vi "Cluster_Analysis.vi"(8 "Shift In":T7[](array[typedef]), 10 "Time Trace in":T6[](array[typedef]), 11 "Analysis Info cluster":T2[](array[typedef]) {"Kurt_u" format="%_3g"; "u^4" format="%_3g"; "u^3" format="%_3g"; "Sd Error in Variance" format="%_3g"; "u^2" format="%_3g"; "Sd Error in Mean" format="%_3g"; "U" format="%_3g"; "Sync Delay Time (s)" format="%.4f"; "Total Meas Time (s)" format="%_5g"; "Skew_u" format="%_3g"; "% u'/U" format="%_3g"}) -> (0 "Shift Out":T7[](array[typedef]), 1 "Autocorrelation":T1[](array[typedef]) {"X array" format="%^_5g"; "Y array" format="%^_5g"}, 2 "Histogram":T1[](array[typedef]) {"X array" format="%^_5g"; "Y array" format="%^_5g"}, 3 "Analysis Info Cluster Out":T2[](array[typedef]) {"Kurt_u" format="%_3g"; "u^4" format="%_3g"; "u^3" format="%_3g"; "Sd Error in Variance" format="%_3g"; "u^2" format="%_3g"; "Sd Error in Mean" format="%_3g"; "U" format="%_3g"; "Sync Delay Time (s)" format="%.4f"; "Total Meas Time (s)" format="%_5g"; "Skew_u" format="%_3g"; "% u'/U" format="%_3g"}, 4 "Spectra":T1[](array[typedef]) {"X array" format="%^_5g"; "Y array" format="%^_5g"}, 5 "Error String":string)   [LabVIEW 2022 SP3]
uses:
  Controls/Shift_Cluster.ctl
  Controls/Time_Trace_Cluster.ctl
  Controls/Analysis_info_cluster.ctl
  Controls/Inst_type.ctl
  Controls/Instrument_Array.ctl
  Controls/channelState.ctl
  Controls/XY_Plot_Cluster.ctl
  FFID/FFID Calib Constants index.ctl
  Globals/Meas_global.vi
  Globals/LDA_global.vi
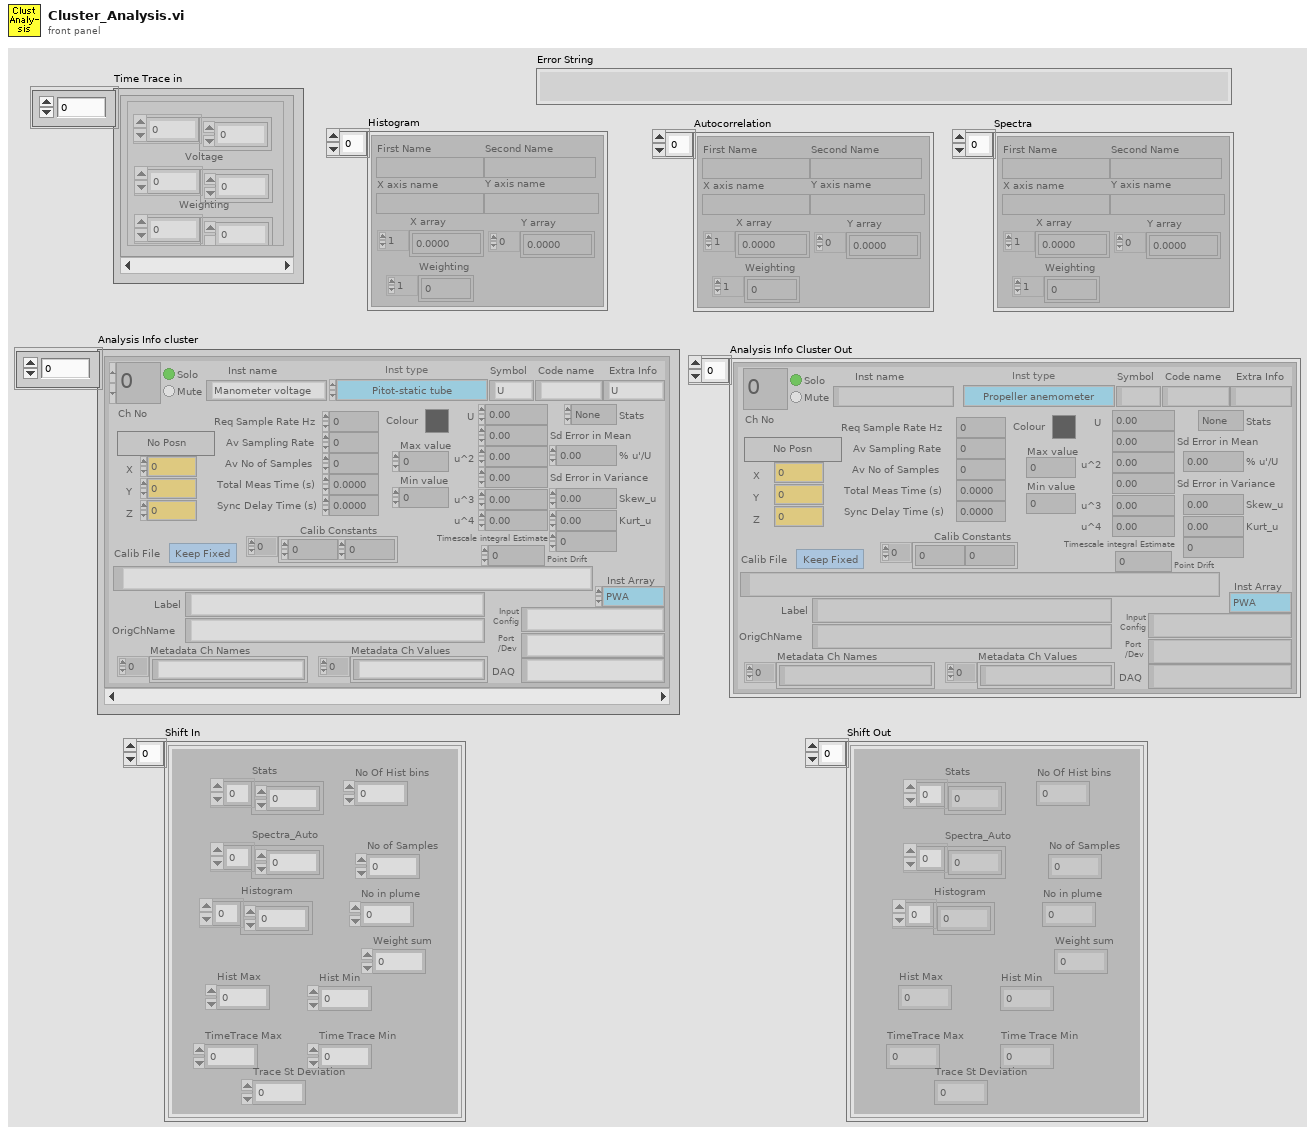
[diagram p1: front panel]
types:
  T1 = typedef "XY_Plot_Cluster.ctl" = cluster{"First Name":string, "Second Name":string, "X axis name":string, "Y axis name":string, "X array":dbl[], "Y array":dbl[], "Weighting":dbl[]}
  T2 = typedef "Analysis_info_cluster.ctl" = cluster{"Colour":u32, "Inst type":T3, "Inst name":string, "Symbol":string, "Code name":string, "Extra Info":string, "Inst Array":T4, "U":dbl, "u^2":dbl, "u^3":dbl, "u^4":dbl, "Skew_u":dbl, "Kurt_u":dbl, "Sd Error in Mean":dbl, "% u'/U":dbl, "X":dbl, "Y":dbl, "Z":dbl, "Timescale integral Estimate":dbl, "Sd Error in Variance":dbl, "Calib File":path, "Calib Constants":dbl[], "Output Position":bool, "Stats":enum16{"None", "Basic", "Full"}, "Av Sampling Rate":dbl, "Av No of Samples":dbl, "Total Meas Time (s)":dbl, "OrigChName":string, "Max value":dbl, "Min value":dbl, "Req Sample Rate Hz":dbl, "Sync Delay Time (s)":dbl, "Ch No":i16, "Device":string, "Use Latest Calib":bool, "Port":string, "Metadata Ch Names":string[], "Metadata Ch Values":string[], "Label":string, "chState":T5, "Point Drift":dbl, "inputConfig":string}
  T3 = typedef "Inst_type.ctl" = enum16{"Raw voltage", "Raw with zero offsetting", "Propeller anemometer", "Pressure Transducer", "Pitot-static tube", "Hot wire", "Cross wire 1", "Cross wire 2", "Generic Linear", "Generic Polynomial", "Generic BackPoly", "Fast FID", "Thermocouple", "Cold wire", "Pulsed Wire", "LDA Vel", "LDA Tran time", "LDA Arr time", "Microphone"}
  T4 = typedef "Instrument_Array.ctl" = enum16{"PWA", "LDA", "Analogue"}
  T5 = typedef "channelState.ctl" = enum32{"No Selection", "Solo", "Mute"}
  T6 = typedef "Time_Trace_Cluster.ctl" = cluster{"Weighting":dbl[], "Voltage":dbl[], "Eng Values":dbl[]}
  T7 = typedef "Shift_Cluster.ctl" = cluster{"Stats":dbl[], "Spectra_Auto":dbl[], "Histogram":dbl[], "Hist Max":dbl, "Hist Min":dbl, "No of Samples":i32, "No in plume":i32, "Weight sum":dbl, "No Of Hist bins":i32, "TimeTrace Max":dbl, "Time Trace Min":dbl, "Trace St Deviation":dbl}
  T8 = typedef "FFID Calib Constants index.ctl" = u16
  T9 = typedef "LDA_Channel.ctl" = cluster{"Wavelength (nm)":dbl, "Vel Comp":string, "Max Velocity":dbl, "Min Velocity":dbl, "Max Record length":u16, "Signal gain (dB)":i16, "High voltage":i16, "Optics Conversion Factor":dbl, "Min Record length":u16, "Multiply Velocity by -1":bool, "Signal to Noise Ratio":string, "Validation Ratio":string, "Probe":string, "Laser":string, "BSA":string, "Lense":string, "Beam Separation (mm)":dbl, "Focal Length (mm)":dbl, "COLOUR":u32, "BSA IP":string, "Velocity Range (m/s)":dbl, "Centre Velocity (m/s)":dbl, "Unshifted mW":dbl, "Shifted mW":dbl, "Bandwidth Hz":dbl, "Req Sampling Rate Hz":dbl, "Ch":i32, "CenterFreq Hz":dbl, "Laser IP":string, "Sync Delay (s)":dbl}
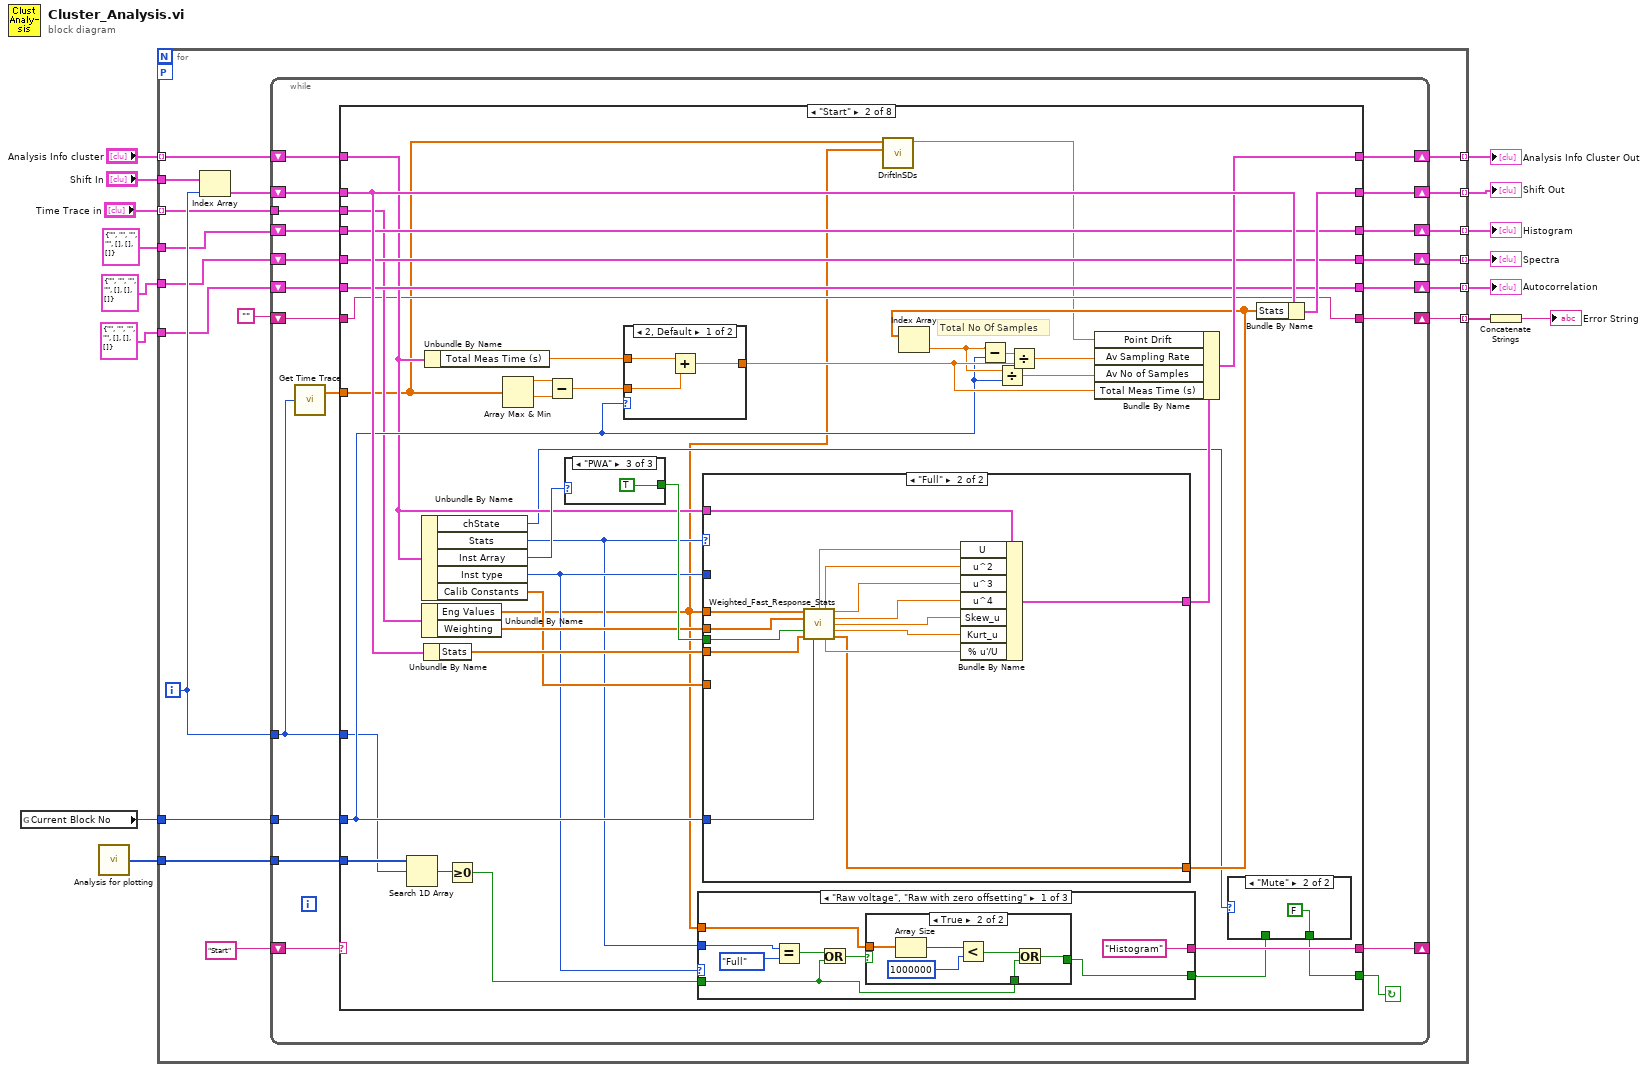
[diagram p0: block diagram]
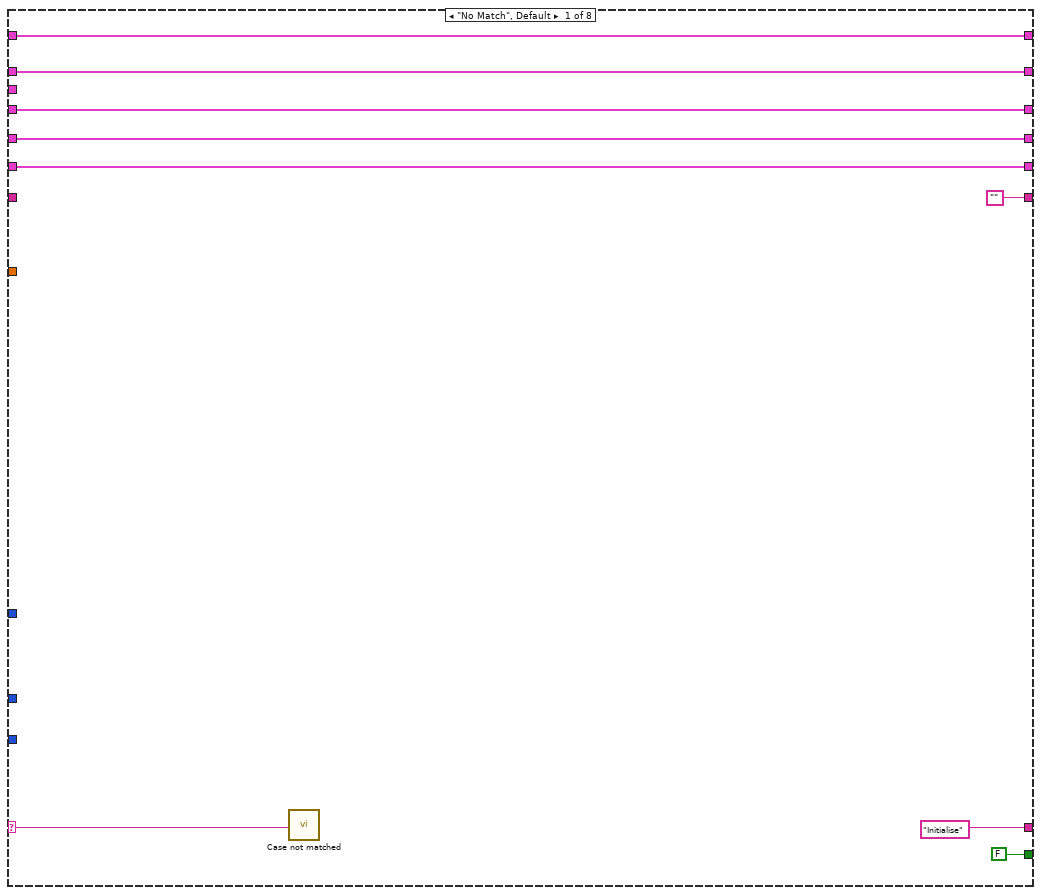
[diagram p2: hidden frame]
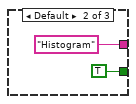
[diagram p5: hidden frame]
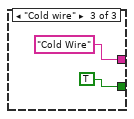
[diagram p6: hidden frame]
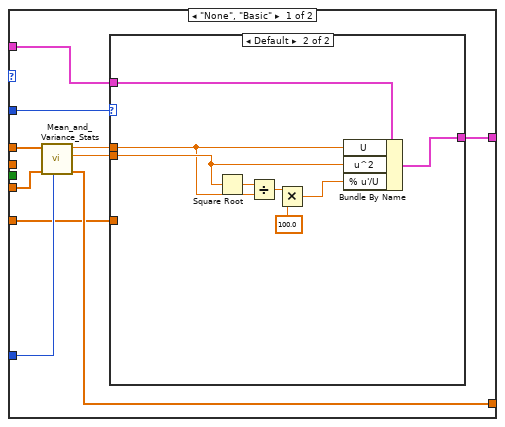
[diagram p8: hidden frame]
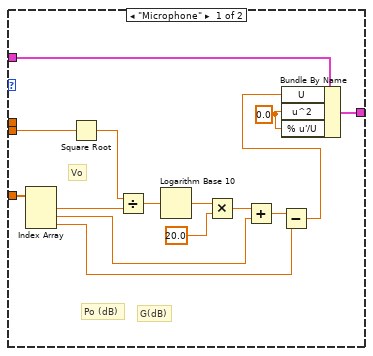
[diagram p9: hidden frame]
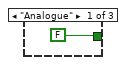
[diagram p10: hidden frame]
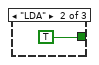
[diagram p11: hidden frame]
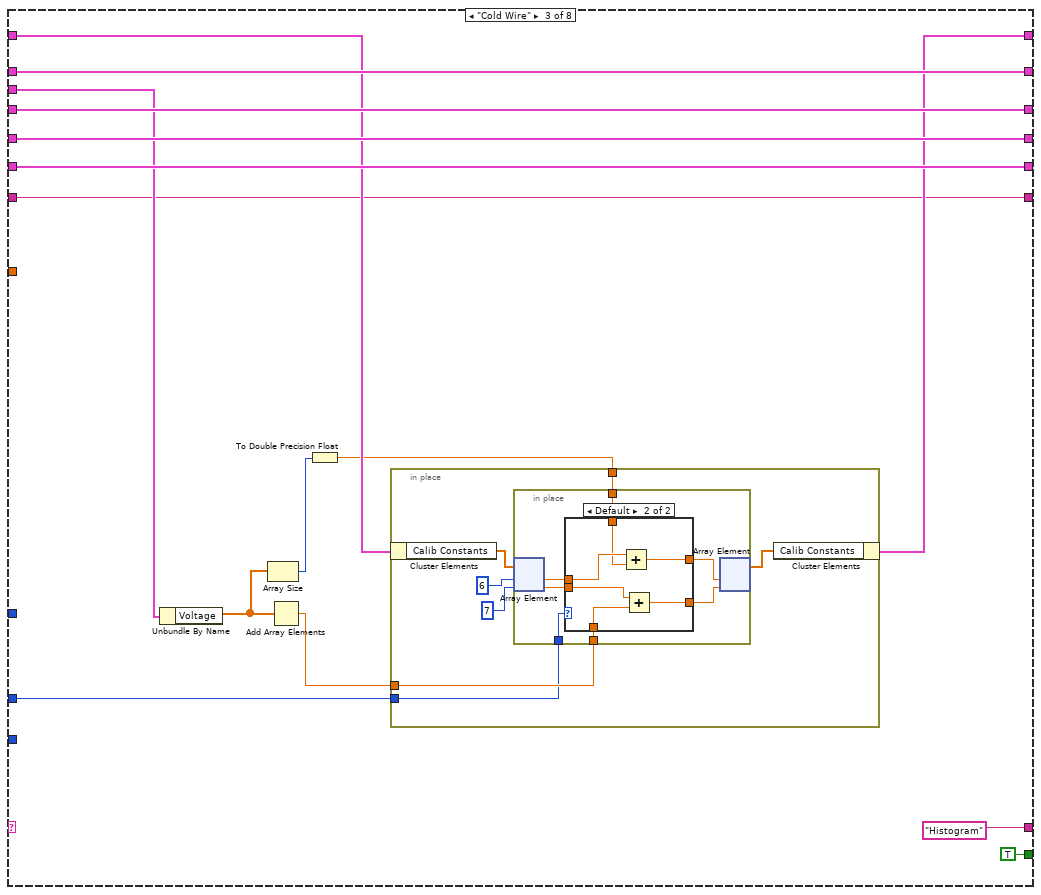
[diagram p12: hidden frame]
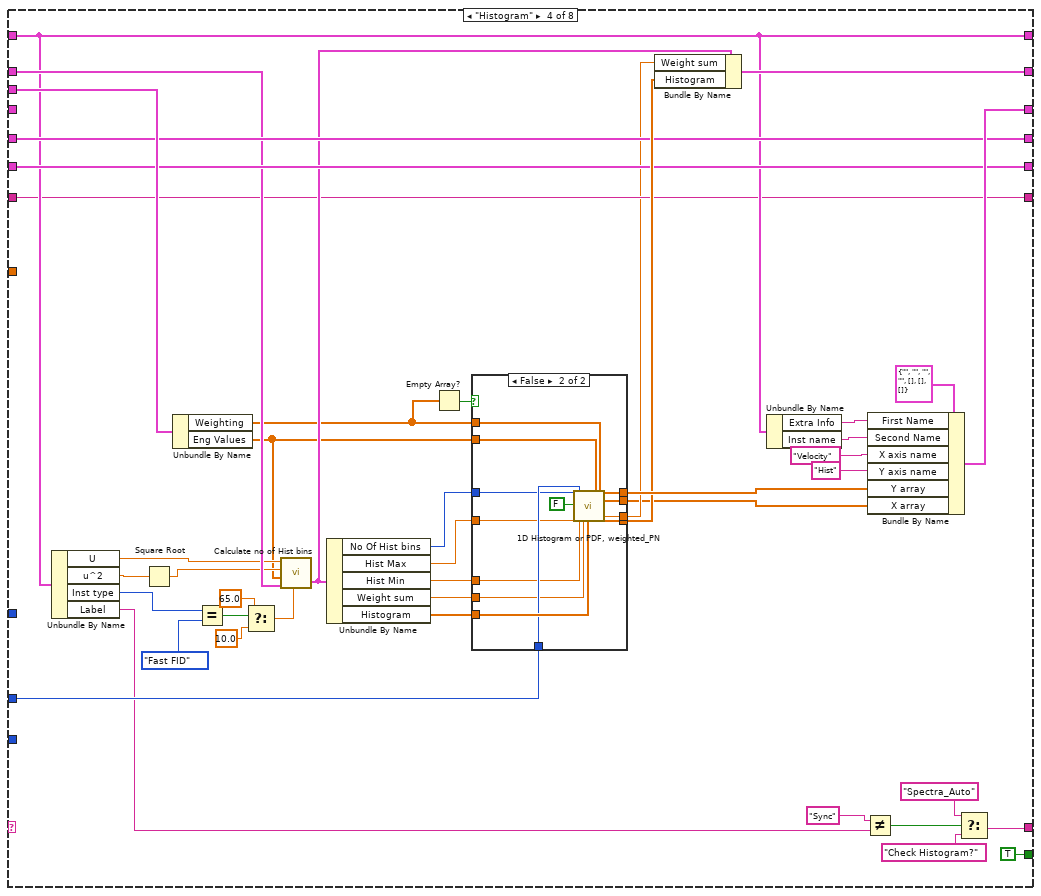
[diagram p14: hidden frame]
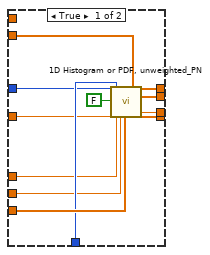
[diagram p15: hidden frame]
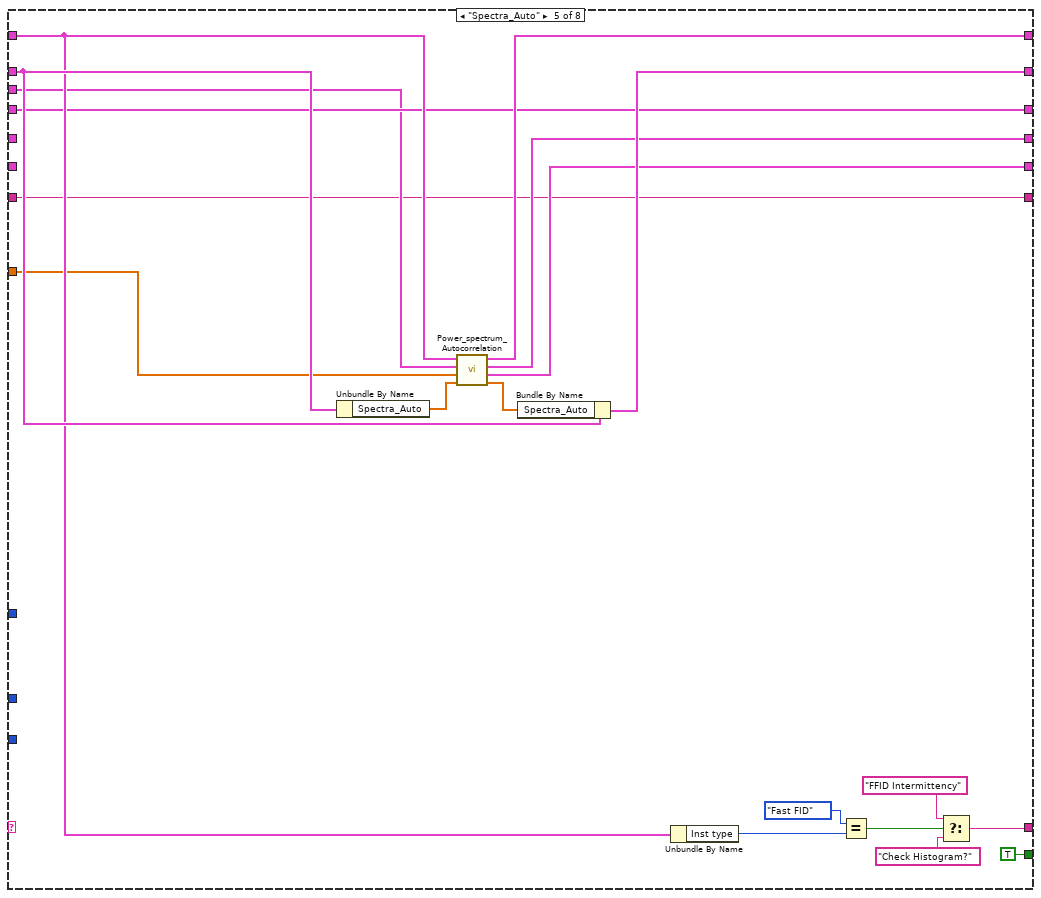
[diagram p16: hidden frame]
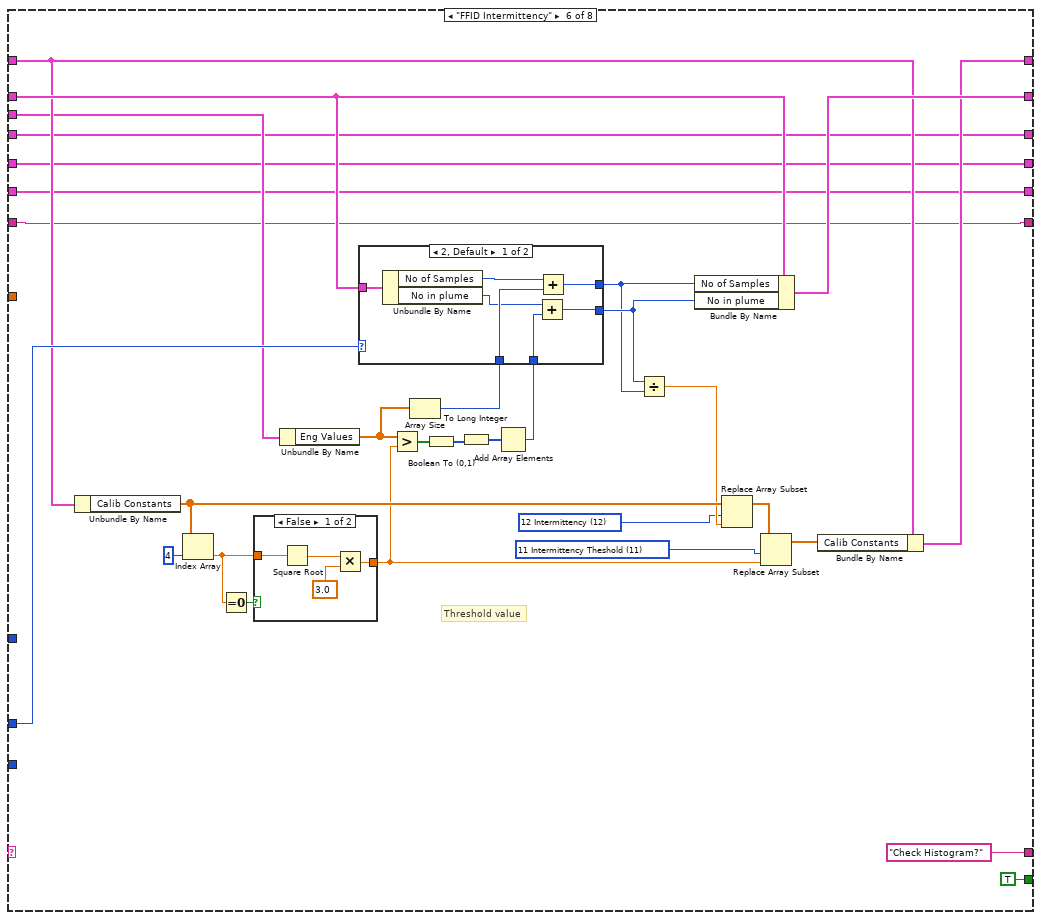
[diagram p17: hidden frame]
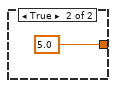
[diagram p19: hidden frame]
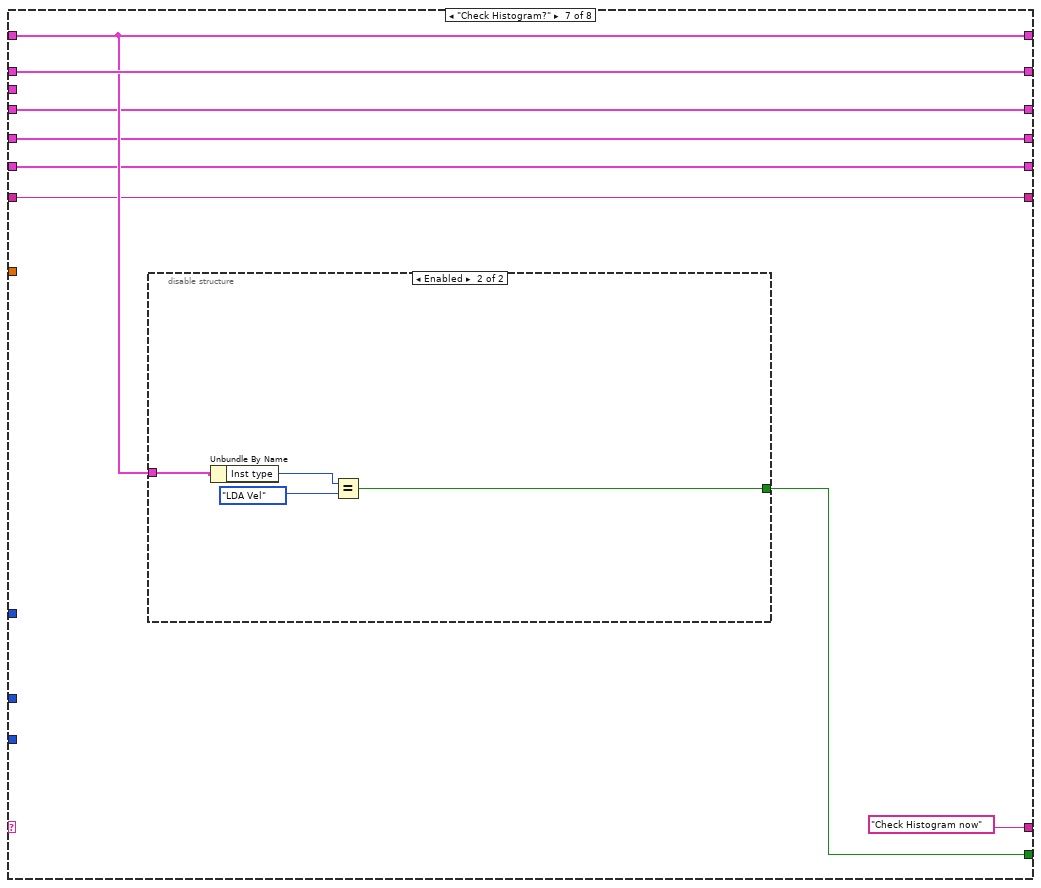
[diagram p20: hidden frame]
diagram:
  n1 = global read "Meas_global.vi" "Current Block No"() -> (w5:i32)
  n2 = call "Analysis for plotting.vi"() -> ("Index of Hist and Spec"=w1:i32[])  [unwired: 5 in]
  n3 = for {
    tunnel: "Shift In" -> [w32]
    tunnel: "Analysis Info cluster" -> [w25] mode=indexing
    tunnel: [w30] -> w14 mode=indexing
    tunnel: [w29] -> w13 mode=indexing
    tunnel: "Time Trace in" -> [w22] mode=indexing
    tunnel: [w28] -> w12 mode=indexing
    tunnel: [w27] -> w10 mode=indexing
    tunnel: [w26] -> w11 mode=indexing
    tunnel: [w24] -> w9 mode=indexing
    tunnel: w5 -> [w21]
    workers-P: _ -> [_]
    tunnel: T1 {"First Name"="", "Second Name"="", "X axis name"="", "Y axis name"="", "X array"=[], "Y array"=[], "Weighting"=[]} ("element") -> [w20]
    tunnel: T1 {"First Name"="", "Second Name"="", "X axis name"="", "Y axis name"="", "X array"=[], "Y array"=[], "Weighting"=[]} ("Spectra") -> [w19]
    tunnel: T1 {"First Name"="", "Second Name"="", "X axis name"="", "Y axis name"="", "X array"=[], "Y array"=[], "Weighting"=[]} ("Autocorrelation") -> [w18]
    tunnel: w1 -> [w16]
    i -> [w23]
    n4 = Index Array(array=w32, index=w23) -> (element=w31:T7)
    n5 = while {
      shift-left: "Start" -> [w51]
      shift-right: [w52] -> _
      shift-right: [w49] -> w29
      shift-left: w25 -> [w50]
      shift-right: [w47] -> w30
      shift-left: w31 -> [w48]
      tunnel: w22 -> [w46]
      shift-right: [w44] -> w28
      shift-left: w20 -> [w45]
      shift-right: [w43] -> w27
      shift-left: w19 -> [w41]
      shift-right: [w42] -> w26
      shift-left: w18 -> [w40]
      shift-right: [w39] -> w24
      shift-left: "" -> [w38]
      tunnel: w23 -> [w37]
      tunnel: w21 -> [w36]
      tunnel: w16 -> [w34]
      stop <- w53 continue-if-true
      n6 = call "Get Time Trace.vi"("Channel Index"=w37) -> ("Time (s)"=w35:dbl[])  [unwired: 1 out]
      n7 = case shown="\"Start\"" w51 {
        selector: w51 -> [w54 _ _ _ _ _ _ _]
        tunnel: [FALSE w67 TRUE ("Processing last block?") TRUE ("Processing last block?") TRUE ("Processing last block?") TRUE ("Full Stats") w347 FALSE ("Processing last block?")] -> w53
        tunnel: ["Initialise" w74 "Histogram" w250 w291 "Check Histogram?" "Check Histogram now" ("f") "End" ("f")] -> w52
        tunnel: w50 -> [w60 w79 w184 w236 w296 w319 w352 w381]
        tunnel: [w60 w93 w183 w236 w299 w318 w352 w381] -> w49
        tunnel: w48 -> [w59 w99 w192 w237 w301 w331 w353 w388]
        tunnel: [w59 w97 w192 w257 w300 w330 w353 w388] -> w47
        tunnel: w36 -> [_ w86 w180 w243 _ w324 _ _]
        tunnel: w46 -> [_ w77 w186 w242 w288 w311 _ _]
        tunnel: w45 -> [w58 w84 w191 _ w289 w309 w350 w380]
        tunnel: [w58 w84 w191 w241 w289 w309 w350 w380] -> w44
        tunnel: [w57 w82 w190 w239 w287 w308 w349 w377] -> w43
        tunnel: [w56 w83 w189 w238 w286 w307 w348 w376] -> w42
        tunnel: w41 -> [w57 w82 w190 w239 _ w308 w349 w377]
        tunnel: w40 -> [w56 w83 w189 w238 _ w307 w348 w376]
        tunnel: ["" w76 w178 w222 w284 w304 w346 w375] -> w39
        tunnel: w38 -> [_ w76 w178 w222 w284 w304 w346 _]
        tunnel: w37 -> [_ w71 _ _ _ _ _ w373]
        tunnel: w35 -> [_ w65 _ _ w283 _ _ _]
        tunnel: w34 -> [_ w72 _ _ _ _ _ _]
        frame "No Match", Default {
          n8 = call "Case not matched.vi"("Case Name not Matched"=w54) -> ()
        }
        frame "Start" {
          # "Total No Of Samples"
          n9 = Search 1D Array(1D array=w72, element=w71) -> (index of element=w70:i32)  [unwired: 1 in]
          n10 = Unbundle By Name(w79) -> ("chState"=w68:T5, "Stats"=w73:enum16{"None", "Basic", "Full"}, "Inst Array"=w101:T4, "Inst type"=w75:T3, "Calib Constants"=w80:dbl[])
          n11 = Unbundle By Name(w77) -> ("Eng Values"=w64:dbl[], "Weighting"=w85:dbl[])
          n12 = Unbundle By Name(w99) -> ("Stats"=w98:dbl[])
          n13 = Unbundle By Name(w79) -> ("Total Meas Time (s)"=w78:dbl)
          n14 = Greater Or Equal To 0?(x=w70) -> (x >= 0?=w69:bool)
          n15 = Array Max & Min(array=w65) -> (max value=w96:dbl, min value=w95:dbl)  [unwired: 2 out]
          n16 = Subtract(x=w96, y=w95) -> (x-y=w81:dbl)
          n17 = case shown="\"PWA\"" w101 {
            tunnel: [FALSE TRUE TRUE] -> w100
            frame "Analogue" {
            }
            frame "LDA" {
            }
            frame "PWA" {
            }
          }
          n18 = case shown="2, Default" w86 {
            tunnel: w81 -> [w125 w126]
            tunnel: w78 -> [w124 _]
            tunnel: [w123 w126] -> w90
            frame 2, Default {
              n19 = Add(x=w124, y=w125) -> (x+y=w123:dbl)
            }
            frame 1 {
            }
          }
          n20 = case shown="\"Raw voltage\", \"Raw with zero offsetting\"" w75 {
            tunnel: [w107 TRUE ("Processing last block?") TRUE ("Processing last block?")] -> w66
            tunnel: ["Histogram" "Histogram" "Cold Wire"] -> w74
            tunnel: w73 -> [w110 _ _]
            tunnel: w64 -> [w108 _ _]
            tunnel: w69 -> [w104 _ _]
            frame "Raw voltage", "Raw with zero offsetting" {
              n21 = Equal?(x=w110, y=enum16{"None", "Basic", "Full"}."Full" ("Stats")) -> (x = y?=w105:bool)
              n22 = Or(x=w105, y=w104) -> (x .or. y?=w106:bool)
              n23 = case shown="True" w106 {
                selector: w106 -> [w112 _]
                tunnel: w108 -> [_ w118]
                tunnel: [w112 w115] -> w107
                tunnel: w104 -> [_ w113]
                frame False {
                }
                frame True {
                  n24 = Array Size(array=w118) -> (size(s)=w117:i32)
                  n25 = Less?(x=w117, y=1000000) -> (x < y?=w114:bool)
                  n26 = Or(x=w114, y=w113) -> (x .or. y?=w115:bool)
                }
              }
            }
            frame Default {
            }
            frame "Cold wire" {
            }
          }
          n27 = case shown="\"Full\"" w73 {
            tunnel: w85 -> [_ w167]
            tunnel: w64 -> [w136 w166]
            tunnel: w100 -> [_ w165]
            tunnel: w79 -> [w134 w164]
            tunnel: w98 -> [w132 w163]
            tunnel: [w131 w162] -> w92
            tunnel: [w133 w161] -> w94
            tunnel: w86 -> [w135 w160]
            tunnel: w75 -> [w128 _]
            tunnel: w80 -> [w127 _]
            frame "None", "Basic" {
              n28 = call "Mean_and_Variance_Stats.vi"("Block No"=w135, "Shift in"=w132, "U"=w136) -> ("Shift out"=w131:dbl[], "u^2"=w130:dbl, "U"=w129:dbl)  [unwired: 3 in]
              n29 = case shown="Default" w128 {
                tunnel: w134 -> [w151 w159]
                tunnel: [w150 w158] -> w133
                tunnel: w130 -> [w149 w157]
                tunnel: w129 -> [_ w155]
                tunnel: w127 -> [w139 _]
                frame "Microphone" {
                  w148 = 0.0 ("u^2")
                  # "Po (dB)"
                  # "G(dB)"
                  # "Vo"
                  n30 = Index Array(array=w139) -> (element #1=w140:dbl, element #2=w145:dbl, element #3=w147:dbl)  [unwired: 3 in]
                  n31 = Square Root(x=w149) -> (sqrt(x)=w138:dbl)
                  n32 = Divide(x=w138, y=w140) -> (x/y=w141:dbl)
                  n33 = Logarithm Base 10(1:w141) -> (0:w142:dbl)
                  n34 = Multiply(x=w142, y=20.0) -> (x*y=w144:dbl)
                  n35 = Add(x=w144, y=w145) -> (x+y=w146:dbl)
                  n36 = Subtract(x=w146, y=w147) -> (x-y=w137:dbl)
                  n37 = Bundle By Name(cluster=w151, "U"=w137, "u^2"=w148, "% u'/U"=w148) -> (w150:T2)
                }
                frame Default {
                  n38 = Square Root(x=w157) -> (sqrt(x)=w156:dbl)
                  n39 = Divide(x=w156, y=w155) -> (x/y=w154:dbl)
                  n40 = Multiply(x=w154, y=100.0) -> (x*y=w152:dbl)
                  n41 = Bundle By Name(cluster=w159, "U"=w155, "u^2"=w157, "% u'/U"=w152) -> (w158:T2)
                }
              }
            }
            frame "Full" {
              n42 = call "Weighted_Fast_Response_Stats.vi"("U"=w166, "Weighting"=w167, "Use Weighting?"=w165, "Shift in"=w163, "Block No"=w160) -> ("U"=w168:dbl, "u^2"=w169:dbl, "u^3"=w170:dbl, "u^4"=w171:dbl, "Skew"=w172:dbl, "Kurt"=w173:dbl, "% u'/U"=w174:dbl, "Shift out"=w162:dbl[])  [unwired: 3 in]
              n43 = Bundle By Name(cluster=w164, "U"=w168, "u^2"=w169, "u^3"=w170, "u^4"=w171, "Skew_u"=w172, "Kurt_u"=w173, "% u'/U"=w174) -> (w161:T2)
            }
          }
          n44 = call "DriftInSDs.vi"("Y"=w64, "X"=w65) -> ("SDratioChange"=w63:dbl)  [unwired: 9 in]
          n45 = Index Array(array=w92) -> (element=w88:dbl)  [unwired: 1 in]
          n46 = Subtract(x=w88, y=w86) -> (x-y=w87:dbl)
          n47 = Divide(x=w88, y=w86) -> (x/y=w89:dbl)
          n48 = Divide(x=w87, y=w90) -> (x/y=w91:dbl)
          n49 = Bundle By Name(cluster=w94, "Point Drift"=w63, "Av Sampling Rate"=w91, "Av No of Samples"=w89, "Total Meas Time (s)"=w90) -> (w93:T2)
          n50 = case shown="\"Mute\"" w68 {
            tunnel: [w102 FALSE ("Processing last block?")] -> w67
            tunnel: w66 -> [w102 _]
            frame Default {
            }
            frame "Mute" {
            }
          }
          n51 = Bundle By Name(cluster=w99, "Stats"=w92) -> (w97:T7)
        }
        frame "Cold Wire" {
          n52 = Unbundle By Name(w186) -> ("Voltage"=w185:dbl[])
          n53 = Array Size(array=w185) -> (size(s)=w182:i32)
          n54 = Add Array Elements(numeric array=w185) -> (sum=w181:dbl)
          n55 = To Double Precision Float(number=w182) -> (double precision float=w179:dbl)
          n56 = in-place {
            in-place-border: w179 -> [w196]
            in-place-border: w181 -> [w195]
            in-place-border: w180 -> [w194]
            n57 = in-place-cluster #1(w184) -> ("Calib Constants"=w199:dbl[])
            n58 = in-place {
              in-place-border: w196 -> [w202]
              in-place-border: w195 -> [w201]
              in-place-border: w194 -> [w200]
              n59 = in-place-array #2(w199, 6, 7) -> (w206:dbl, w204:dbl)
              n60 = case shown="Default" w200 {
                tunnel: w206 -> [_ w214]
                tunnel: [w208 w213] -> w205
                tunnel: w204 -> [_ w212]
                tunnel: [w207 w211] -> w203
                tunnel: w202 -> [w208 w210]
                tunnel: w201 -> [w207 w209]
                frame 1 {
                }
                frame Default {
                  n61 = Add(x=w214, y=w210) -> (x+y=w213:dbl)
                  n62 = Add(x=w212, y=w209) -> (x+y=w211:dbl)
                }
              }
              n63 = in-place-array #2(w205, w203) -> (w198:dbl[])  [unwired: 2 out]
            }
            n64 = in-place-cluster #1("Calib Constants"=w198) -> (w183:T2)
          }
        }
        frame "Histogram" {
          n65 = Unbundle By Name(w236) -> ("U"=w230:dbl, "u^2"=w231:dbl, "Inst type"=w228:T3, "Label"=w221:string)
          n66 = Square Root(x=w231) -> (sqrt(x)=w229:dbl)
          n67 = Unbundle By Name(w242) -> ("Weighting"=w217:dbl[], "Eng Values"=w215:dbl[])
          n68 = Equal?(x=w228, y=Inst_type."Fast FID" ("Inst type")) -> (x = y?=w226:bool)
          n69 = Select(t=65.0, s=w226, f=10.0) -> (s? t:f=w223:dbl)
          n70 = call "Calculate no of Hist bins.vi"("Mean"=w230, "Standard Deviation"=w229, "Time Trace"=w215, "Shift Input"=w237, "Number of Bins per Sigma"=w223) -> ("Shift Output"=w235:T7)  [unwired: 1 in]
          n71 = Unbundle By Name(w235) -> ("No Of Hist bins"=w232:i32, "Hist Max"=w234:dbl, "Hist Min"=w233:dbl, "Weight sum"=w218:dbl, "Histogram"=w246:dbl[])
          n72 = Empty Array?(array=w217) -> (empty?=w216:bool)
          n73 = case shown="False" w216 {
            tunnel: w246 -> [w269 w282]
            tunnel: [w268 w281] -> w245
            tunnel: [w267 w280] -> w244
            tunnel: w243 -> [w265 w278]
            tunnel: w215 -> [w264 w277]
            tunnel: w234 -> [w263 w276]
            tunnel: w233 -> [w262 w275]
            tunnel: w232 -> [w261 w274]
            tunnel: [w260 w273] -> w220
            tunnel: [w259 w272] -> w219
            tunnel: w218 -> [w258 w271]
            tunnel: w217 -> [_ w270]
            frame True {
              n74 = call "1D Histogram or PDF, unweighted_PN.vi"("Nbins"=w261, "Mean shift"=FALSE, "max"=w263, "Current block no."=w265, "min"=w262, "Shift SumW in"=w258, "Shift PDF in"=w269, "1D data"=w264) -> ("1D histogram or PDF"=w268:dbl[], "bin centre vals."=w259:dbl[], "Shift SumW out"=w260:dbl, "Shift PDF out"=w267:dbl[])  [unwired: 15 in, 1 out]
            }
            frame False {
              n75 = call "1D Histogram or PDF, weighted_PN.vi"("Nbins"=w274, "Mean shift"=FALSE, "max"=w276, "Current block no."=w278, "min"=w275, "Shift SumW in"=w271, "Shift PDF in"=w282, "1D data"=w277, "Weights"=w270) -> ("1D histogram or PDF"=w281:dbl[], "bin centre vals."=w272:dbl[], "Shift SumW out"=w273:dbl, "Shift PDF out"=w280:dbl[])  [unwired: 14 in, 1 out]
            }
          }
          n76 = Bundle By Name(cluster=w235, "Weight sum"=w220, "Histogram"=w244) -> (w257:T7)
          n77 = Unbundle By Name(w236) -> ("Extra Info"=w254:string, "Inst name"=w253:string)
          n78 = Not Equal?(x="Sync", y=w221) -> (x != y?=w247:bool)
          n79 = Bundle By Name(cluster=T1 {"First Name"="", "Second Name"="", "X axis name"="", "Y axis name"="", "X array"=[], "Y array"=[], "Weighting"=[]} ("element"), "First Name"=w254, "Second Name"=w253, "X axis name"="Velocity", "Y axis name"="Hist", "Y array"=w245, "X array"=w219) -> (w241:T1)
          n80 = Select(t="Spectra_Auto", s=w247, f="Check Histogram?") -> (s? t:f=w250:string)
        }
        frame "Spectra_Auto" {
          n81 = Unbundle By Name(w301) -> ("Spectra_Auto"=w298:dbl[])
          n82 = call "Power_spectrum_Autocorrelation.vi"("CompositeArrayIn"=w298, "Time (s)"=w283, "Time Trace"=w288, "AnalysisInfoIn"=w296) -> ("CompositeArrayOut"=w297:dbl[], "Autocorrelation"=w286:T1, "Spectra"=w287:T1, "AnalysisInfoOut"=w299:T2)  [unwired: 1 in]
          n83 = Bundle By Name(cluster=w301, "Spectra_Auto"=w297) -> (w300:T7)
          n84 = Unbundle By Name(w296) -> ("Inst type"=w285:T3)
          n85 = Equal?(x=Inst_type."Fast FID" ("Inst type"), y=w285) -> (x = y?=w294:bool)
          n86 = Select(t="FFID Intermittency", s=w294, f="Check Histogram?") -> (s? t:f=w291:string)
        }
        frame "FFID Intermittency" {
          w303 = T8 12 items=["0 Coeff A", "1 Coeff B", "2 Coeff C", "3 FFID Bkgnd", "4 FFID Bkgnd Variance", "5 FFID Bkgnd Volts", "6 FFID Bkgnd Time", "7 GMU Source ppm/%density", "8 Orig Bkgnd Time", "9 Orig Bknd volts", "10 Orig bkgnd Variance", "11 Intermittency Theshold", "12 Intermittency", "13 Head Temp", "14 Exhaust Temp", "15", "16", "17", "18 Calibration Drift %", "19 Calibration Interval Minutes"] ("FFID")
          w302 = T8 11 items=["0 Coeff A", "1 Coeff B", "2 Coeff C", "3 FFID Bkgnd", "4 FFID Bkgnd Variance", "5 FFID Bkgnd Volts", "6 FFID Bkgnd Time", "7 GMU Source ppm/%density", "8 Orig Bkgnd Time", "9 Orig Bknd volts", "10 Orig bkgnd Variance", "11 Intermittency Theshold", "12 Intermittency", "13 Head Temp", "14 Exhaust Temp", "15", "16", "17", "18 Calibration Drift %", "19 Calibration Interval Minutes"] ("FFID")
          # "Threshold value"
          n87 = Unbundle By Name(w319) -> ("Calib Constants"=w317:dbl[])
          n88 = Index Array(array=w317, index=4 ("Index")) -> (element=w326:dbl)
          n89 = Equal To 0?(x=w326) -> (x = 0?=w327:bool)
          n90 = case shown="False" w327 {
            tunnel: [w342 5.0] -> w314
            tunnel: w326 -> [w341 _]
            frame False {
              n91 = Square Root(x=w341) -> (sqrt(x)=w344:dbl)
              n92 = Multiply(x=w344, y=3.0) -> (x*y=w342:dbl)
            }
            frame True {
            }
          }
          n93 = Unbundle By Name(w311) -> ("Eng Values"=w310:dbl[])
          n94 = Greater?(x=w310, y=w314) -> (0:w325:bool[])
          n95 = Array Size(array=w310) -> (size(s)=w323:i32)
          n96 = Boolean To (0,1)(Boolean=w325) -> (0, 1=w306:i16[])
          n97 = To Long Integer(number=w306) -> (32bit integer=w305:i32[])
          n98 = Add Array Elements(numeric array=w305) -> (sum=w322:i32)
          n99 = case shown="2, Default" w324 {
            tunnel: w331 -> [w338 _]
            tunnel: w323 -> [w336 w339]
            tunnel: w322 -> [w335 w340]
            tunnel: [w334 w340] -> w321
            tunnel: [w333 w339] -> w320
            frame 2, Default {
              n100 = Unbundle By Name(w338) -> ("No of Samples"=w337:i32, "No in plume"=w332:i32)
              n101 = Add(x=w332, y=w335) -> (x+y=w334:i32)
              n102 = Add(x=w337, y=w336) -> (x+y=w333:i32)
            }
            frame 1 {
            }
          }
          n103 = Divide(x=w321, y=w320) -> (x/y=w316:dbl)
          n104 = Bundle By Name(cluster=w331, "No of Samples"=w320, "No in plume"=w321) -> (w330:T7)
          n105 = Replace Array Subset(array=w317, new element=w316, index=w303) -> (w315:dbl[])
          n106 = Replace Array Subset(array=w315, new element=w314, index=w302) -> (w313:dbl[])
          n107 = Bundle By Name(cluster=w319, "Calib Constants"=w313) -> (w318:T2)
        }
        frame "Check Histogram?" {
          n108 = disable-structure shown="Enabled" {
            disable-tunnel: w352 -> [w359 w368]
            disable-tunnel: [w354 w365] -> w347
            frame Disabled {
              n109 = Unbundle By Name(w359) -> ("Inst name"=w357:string)
              n110 = for {
                tunnel: string[] ["RV (WT", "RV (Sync)"] ("appended array") -> [w361] mode=indexing
                tunnel: w357 -> [w364]
                tunnel: [w360] -> w356 mode=indexing
                n111 = String Length(string=w361) -> (length=w363:i32)
                n112 = String Subset(string=w364, length (rest)=w363) -> (substring=w362:string)  [unwired: 1 in]
                n113 = Equal?(x=w361, y=w362) -> (x = y?=w360:bool)
              }
              n114 = Or Array Elements(Boolean array=w356) -> (logical OR=w355:bool)
              n115 = Not(x=w355) -> (.not. x?=w354:bool)
            }
            frame Enabled {
              n116 = Unbundle By Name(w368) -> ("Inst type"=w366:T3)
              n117 = Equal?(x=w366, y=Inst_type."LDA Vel" ("Inst type")) -> (x = y?=w365:bool)
            }
          }
        }
        frame "Check Histogram now" {
          w369 = 0.0 ("Max Velocity")
          # "Underflow"
          # "Overflow"
          # "Min Vel"
          # "Max Vel"
          # "Max"
          # "Hist"
          n118 = global read "Meas_global.vi" "No of bins in histogram"() -> (w385:i32)
          n119 = Unbundle By Name(w381) -> ("Inst name"=w382:string, "Inst type"=w383:T3, "Code name"=w374:string)
          n120 = Unbundle By Name(w380) -> ("X array"=w379:dbl[], "Y array"=w378:dbl[])
          n121 = while {
            tunnel: w385 -> [w406]
            shift-left: w369 -> [w407]
            shift-right: [w409] -> _
            shift-left: dbl[] [] -> [w408]
            shift-right: [w410] -> _
            shift-left: "" -> [w411]
            shift-right: [w412] -> w375
            shift-left: 0 -> [w413]
            shift-right: [w414] -> _
            shift-left: 0 -> [w417]
            shift-right: [w415] -> _
            shift-right: [w403] -> _
            shift-left: w369 -> [w401]
            shift-right: [w402] -> _
            shift-left: w369 -> [w400]
            shift-right: [w399] -> _
            shift-left: w369 -> [w396]
            shift-right: [w398] -> _
            shift-left: w369 -> [w397]
            tunnel: w383 -> [w395]
            tunnel: w379 -> [w394]
            tunnel: w378 -> [w393]
            tunnel: w382 -> [w392]
            tunnel: w381 -> [w391]
            tunnel: w374 -> [w390]
            tunnel: w373 -> [w389]
            stop <- w418 continue-if-true
            n122 = Increment(x=w417) -> (x+1=w416:i32)
            n123 = case shown="7" w417 {
              tunnel: [TRUE TRUE TRUE TRUE TRUE TRUE TRUE w589 TRUE TRUE TRUE TRUE TRUE TRUE FALSE] -> w418
              tunnel: w416 -> [w428 w442 w456 w501 w532 w547 _ w597 w617 w652 w677 w698 w705 w726 w728]
              tunnel: [w428 w443 w454 w503 w532 w555 w581 w597 w617 w652 w679 w698 w707 w726 w728] -> w415
              tunnel: [w423 w445 w469 w489 w524 w538 w576 w599 w624 w659 w680 w694 w708 w722 w730] -> w414
              tunnel: w413 -> [w423 w445 w469 _ w524 _ w576 w599 w624 w659 w680 w694 w708 w722 w730]
              tunnel: ["" w444 w468 w502 w530 w554 w583 w601 w625 w660 w683 w696 w711 w724 w731] -> w412
              tunnel: w411 -> [_ w444 w468 w502 w531 w554 w584 w601 w625 w660 w683 w697 w711 w725 w731]
              tunnel: [w426 w429 w466 w494 w528 w544 w582 w600 w620 w655 w682 w695 w710 w723 w737] -> w410
              tunnel: [w425 w436 w467 w492 w527 w542 w578 w598 w618 w653 w681 w690 w709 w718 w736] -> w409
              tunnel: w408 -> [w426 _ w466 w494 w528 w544 w582 w600 w620 w655 w682 w695 w710 w723 w737]
              tunnel: w407 -> [w425 w436 w467 _ w527 _ w578 _ w618 w653 w681 w690 w709 w718 w736]
              tunnel: w406 -> [_ _ _ w495 _ w551 _ _ w606 w640 _ _ _ _ _]
              tunnel: 7 -> [_ w441 _ _ _ _ _ _ _ _ _ _ _ _ _]
              tunnel: 14 ("y") -> [_ _ w455 _ _ w546 w581 _ _ _ _ _ _ _ _]
              tunnel: [w422 w440 w452 w488 w522 w537 w574 w594 w612 w648 w675 w686 w703 w717 w735] -> w403
              tunnel: [w421 w439 w451 w487 w521 w536 w573 w593 w613 w647 w674 w689 w702 w714 w734] -> w402
              tunnel: w401 -> [w422 w440 w452 w488 w522 w537 w574 _ w612 w648 w675 w686 w703 w717 w735]
              tunnel: w400 -> [w421 w439 w451 w487 w521 w536 w573 _ w613 w647 w674 w689 w702 w714 w734]
              tunnel: [w419 w437 w449 w485 w519 w534 w571 w595 w611 w646 w672 w687 w701 w716 w732] -> w399
              tunnel: [w420 w438 w450 w486 w520 w535 w572 w596 w610 w645 w673 w688 w700 w715 w733] -> w398
              tunnel: w397 -> [w420 w438 w450 w486 w520 w535 w572 w596 w610 _ w673 w688 w700 w715 w733]
              tunnel: w396 -> [w419 w437 w449 w485 w519 w534 w571 w595 _ w646 w672 w687 w701 w716 w732]
              tunnel: w395 -> [_ w435 _ _ _ _ _ _ _ _ _ _ _ _ _]
              tunnel: w394 -> [_ w432 _ _ w517 _ w569 _ w602 w637 _ _ _ _ _]
              tunnel: w393 -> [_ w430 _ _ _ _ _ _ _ _ _ _ _ _ _]
              tunnel: w392 -> [_ _ _ _ w518 _ w570 _ _ _ _ w685 _ w713 _]
              tunnel: w391 -> [_ _ _ _ _ _ _ _ _ _ _ _ _ _ _]
              tunnel: w390 -> [_ _ _ _ _ _ _ w592 _ _ _ _ _ _ _]
              tunnel: w389 -> [_ _ _ _ _ _ _ w586 _ _ _ _ _ _ _]
              frame 0, Default {
              }
              frame 1 {
                n124 = Index Array(array=w432) -> (element #1=w434:dbl, element #2=w433:dbl)  [unwired: 2 in]
                n125 = Subtract(x=w433, y=w434) -> (x-y=w431:dbl)
                n126 = Multiply(x=w431, y=w430) -> (x*y=w429:dbl[])
                n127 = case shown="\"LDA Vel\"" w435 {
                  tunnel: [w447 w448] -> w443
                  tunnel: w442 -> [w447 _]
                  tunnel: w441 -> [_ w448]
                  frame "Propeller anemometer", Default {
                  }
                  frame "LDA Vel" {
                  }
                }
              }
              frame 2 {
                n128 = for {
                  tunnel: w466 -> [w478] mode=indexing
                  shift-right: [w471] -> _
                  shift-left: FALSE -> [w477]
                  shift-right: [w474] -> w460
                  shift-left: 0 -> [w475]
                  shift-right: [w472] -> w462
                  shift-left: 0 -> [w473]
                  n129 = Greater Than 0?(x=w478) -> (x > 0?=w471:bool)
                  n130 = Compound Arithmetic op=AND(w471, invert w477) -> (w476:bool)
                  n131 = case shown="True" w471 {
                    tunnel: w473 -> [w479 w481]
                    tunnel: [w479 w480] -> w472
                    frame False {
                    }
                    frame True {
                      n132 = Increment(x=w481) -> (x+1=w480:i32)
                    }
                  }
                  n133 = case shown="True" w476 {
                    tunnel: w475 -> [w482 w484]
                    tunnel: [w482 w483] -> w474
                    frame False {
                    }
                    frame True {
                      n134 = Increment(x=w484) -> (x+1=w483:i32)
                    }
                  }
                }
                n135 = Equal?(x=w460, y=1) -> (x = y?=w457:bool)
                n136 = Greater?(x=w462, y=10) -> (0:w458:bool)
                n137 = And(x=w458, y=w457) -> (x .and. y?=w453:bool)
                n138 = Select(t=w456, s=w453, f=w455) -> (s? t:f=w454:i32)
              }
              frame 3 {
                # "Clipping?"
                n139 = Increment(x=w495) -> (x+1=w508:i32)
                n140 = while {
                  tunnel: [w509] -> w492
                  tunnel: w494 -> [w516]
                  shift-left: 0.0 -> [w509]
                  shift-right: [w514] -> w505
                  shift-left: w508 -> [w515]
                  shift-right: [w513] -> w491
                  stop <- w510 continue-if-true
                  n141 = Decrement(x=w515) -> (x-1=w513:i32)
                  n142 = Index Array(array=w516, index=w515) -> (element=w514:dbl)
                  n143 = Equal To 0?(x=w509) -> (x = 0?=w511:bool)
                  n144 = Greater Than 0?(x=w513) -> (x > 0?=w512:bool)
                  n145 = And(x=w512, y=w511) -> (x .and. y?=w510:bool)
                }
                n146 = Greater?(x=w492, y=0.04) -> (0:w497:bool)
                n147 = Multiply(x=w492, y=0.7) -> (x*y=w506:dbl)
                n148 = Greater?(x=w506, y=w505) -> (0:w498:bool)
                n149 = Add(x=w491, y=2) -> (x+y=w489:i32)
                n150 = And(x=w497, y=w498) -> (x .and. y?=w496:bool)
                n151 = Increment(x=w501) -> (x+1=w500:i32)
                n152 = Select(t=w501, s=w496, f=w500) -> (s? t:f=w503:i32)
              }
              frame 4 {
                n153 = Multiply(x=w527, y=100.0) -> (x*y=w525:dbl)
                n154 = Index Array(array=w517, index=w524) -> (element=w523:dbl)
                n155 = Format Into String(format string="Histogram of %s may indicate Clipping at Upper limit of %.2f by %.0f%%.\\n" ("Format String"), initial string=w531, w518, w523, w525) -> (resulting string=w530:string)  [unwired: 1 in, 1 out]
              }
              frame 5 {
                # "Clipping?"
                n156 = while {
                  tunnel: w551 -> [w561]
                  tunnel: [w563] -> w542
                  tunnel: w544 -> [w568]
                  shift-left: 0.0 -> [w563]
                  shift-right: [w566] -> w557
                  shift-left: 0 -> [w567]
                  shift-right: [w562] -> w540
                  stop <- w564 continue-if-true
                  n157 = Increment(x=w567) -> (x+1=w562:i32)
                  n158 = Index Array(array=w568, index=w567) -> (element=w566:dbl)
                  n159 = Less?(x=w562, y=w561) -> (x < y?=w560:bool)
                  n160 = Equal To 0?(x=w563) -> (x = 0?=w565:bool)
                  n161 = And(x=w560, y=w565) -> (x .and. y?=w564:bool)
                }
                n162 = Array Max & Min(array=w544) -> (max value=w543:dbl)  [unwired: 3 out]
                n163 = Not Equal?(x=w542, y=w543) -> (x != y?=w541:bool)
                n164 = Greater?(x=w542, y=0.04) -> (0:w549:bool)
                n165 = Multiply(x=w542, y=0.45) -> (x*y=w558:dbl)
                n166 = Greater?(x=w558, y=w557) -> (0:w550:bool)
                n167 = Subtract(x=w540, y=2) -> (x-y=w538:i32)
                n168 = Compound Arithmetic op=AND(w541, w549, w550) -> (w548:bool)
                n169 = Select(t=w547, s=w548, f=w546) -> (s? t:f=w555:i32)
              }
              frame 6 {
                n170 = Index Array(array=w569, index=w576) -> (element=w575:dbl)
                n171 = Multiply(x=w578, y=100.0) -> (x*y=w577:dbl)
                n172 = Format Into String(format string="Histogram of %s may indicate Clipping at Lower limit of %.2f by %.0f%%.\\n" ("Format String"), initial string=w584, w570, w575, w577) -> (resulting string=w583:string)  [unwired: 1 in, 1 out]
              }
              frame 7 {
                n173 = global read "LDA_global.vi" "LDA Channels"() -> (w588:T9[])
                n174 = Match Pattern(string=w592, regular expression="Derived") -> (offset past match=w590:i32)  [unwired: 1 in, 3 out]
                n175 = Index Array(array=w588, index=w586) -> (element=w587:T9)
                n176 = Less Than 0?(x=w590) -> (x < 0?=w589:bool)
                n177 = Unbundle By Name(w587) -> ("Max Velocity"=w594:dbl, "Min Velocity"=w593:dbl)
                n178 = Add Array Elements(numeric array=w600) -> (sum=w598:dbl)
              }
              frame 8 {
                n179 = Divide(x=w606, y=2) -> (x/y=w604:dbl)
                n180 = Array Max & Min(array=w602) -> (max value=w609:dbl, min value=w608:dbl)  [unwired: 2 out]
                n181 = Subtract(x=w609, y=w608) -> (x-y=w607:dbl)
                n182 = Divide(x=w607, y=w604) -> (x/y=w603:dbl)
                n183 = Subtract(x=w612, y=w603) -> (x-y=w623:dbl)
                n184 = for {
                  tunnel: w623 -> [w630]
                  shift-right: [w628] -> w619
                  shift-left: 0.0 -> [w631]
                  tunnel: w620 -> [w632] mode=indexing
                  tunnel: w602 -> [w627] mode=indexing
                  n185 = Greater?(x=w627, y=w630) -> (0:w629:bool)
                  n186 = case shown="True" w629 {
                    tunnel: w632 -> [_ w635]
                    tunnel: w631 -> [w633 w636]
                    tunnel: [w633 w634] -> w628
                    frame False {
                    }
                    frame True {
                      n187 = Add(x=w635, y=w636) -> (x+y=w634:dbl)
                    }
                  }
                }
                n188 = Divide(x=w619, y=w618) -> (x/y=w615:dbl)
                n189 = Greater?(x=w615, y=0.025) -> (0:w616:bool)
                n190 = Select(t=w615, s=w616, f=0.0) -> (s? t:f=w611:dbl)
              }
              frame 9 {
                n191 = Array Max & Min(array=w637) -> (max value=w644:dbl, min value=w643:dbl)  [unwired: 2 out]
                n192 = Divide(x=w640, y=2) -> (x/y=w639:dbl)
                n193 = Subtract(x=w644, y=w643) -> (x-y=w642:dbl)
                n194 = Divide(x=w642, y=w639) -> (x/y=w638:dbl)
                n195 = Add(x=w647, y=w638) -> (x+y=w658:dbl)
                n196 = for {
                  tunnel: w658 -> [w665]
                  shift-right: [w663] -> w654
                  shift-left: 0.0 -> [w666]
                  tunnel: w655 -> [w667] mode=indexing
                  tunnel: w637 -> [w662] mode=indexing
                  n197 = Less?(x=w662, y=w665) -> (x < y?=w664:bool)
                  n198 = case shown="True" w664 {
                    tunnel: w667 -> [_ w670]
                    tunnel: w666 -> [w668 w671]
                    tunnel: [w668 w669] -> w663
                    frame False {
                    }
                    frame True {
                      n199 = Add(x=w670, y=w671) -> (x+y=w669:dbl)
                    }
                  }
                }
                n200 = Divide(x=w654, y=w653) -> (x/y=w650:dbl)
                n201 = Greater?(x=w650, y=0.025) -> (0:w651:bool)
                n202 = Select(t=w650, s=w651, f=0.0) -> (s? t:f=w645:dbl)
              }
              frame 10 {
                n203 = Equal To 0?(x=w672) -> (x = 0?=w678:bool)
                n204 = Increment(x=w677) -> (x+1=w676:i32)
                n205 = Select(t=w676, s=w678, f=w677) -> (s? t:f=w679:i32)
              }
              frame 11 {
                n206 = Multiply(x=w687, y=100.0) -> (x*y=w691:dbl)
                n207 = Format Into String(format string="%.1f %% of the %s samples are too close to the upper velocity limit of %.2f m/s.\n" ("Format String"), initial string=w697, w691, w685, w686) -> (resulting string=w696:string)  [unwired: 1 in, 1 out]
              }
              frame 12 {
                n208 = Increment(x=w705) -> (x+1=w704:i32)
                n209 = Equal To 0?(x=w700) -> (x = 0?=w706:bool)
                n210 = Select(t=w704, s=w706, f=w705) -> (s? t:f=w707:i32)
              }
              frame 13 {
                n211 = Multiply(x=w715, y=100.0) -> (x*y=w719:dbl)
                n212 = Format Into String(format string="%.1f %% of the %s samples are too close to the lower velocity limit of %.2f m/s.\n" ("Format String"), initial string=w725, w719, w713, w714) -> (resulting string=w724:string)  [unwired: 1 in, 1 out]
              }
              frame 14 {
              }
            }
          }
        }
      }
    }
  }
  "Shift Out" <- w14
  "Analysis Info Cluster Out" <- w13
  "Histogram" <- w12
  "Spectra" <- w10
  "Autocorrelation" <- w11
  n213 = Concatenate Strings(w9) -> (→"Error String":string)
